vi "V_Estados.vi"() -> ()   [LabVIEW 2022 SP3]
uses:
  <vilib>/imath/engines/lvmath2/RunTimeEngine/Managers/WorkSpace/UID Generator.vi
  <vilib>/imath/engines/lvmath2/RunTimeEngine/RunTimeType/NIMS_RunTimeType_From StrictType (excl LVString).vi
  <instcachedir>/0/NIMS_RunTimeType_From StrictType (excl LVString)_70DEE8F51B6B495C85F505DE4E7061F1.lvgen/NIMS_RunTimeType_From StrictType (excl LVString)_70DEE8F51B6B495C85F505DE4E7061F1_000.vi
  <vilib>/imath/engines/lvmath2/RunTimeEngine/LocalVariableDefStatement/MC_LocalVariableDefStatement_Display.vi
  <vilib>/imath/engines/lvmath2/RunTimeEngine/VariableToken/NIMS_VariableToken_CondDefined.vi
  <instcachedir>/0/NIMS_VariableToken_CondDefined_190C34D11DD44198A50DB545329B6163.lvgen/NIMS_VariableToken_CondDefined_190C34D11DD44198A50DB545329B6163_003.vi
  <vilib>/imath/engines/lvmath2/RunTimeEngine/BuiltInFunctions/tf_to_ss/NIMS_tf_to_ss.vi
  <vilib>/imath/engines/lvmath2/RunTimeEngine/ErrorHandling/NIMS_Create Error From Enums.vi
  <vilib>/imath/engines/lvmath2/RunTimeEngine/BuiltInFunctions/transpose/NIMS_transpose(GM).vi
  <instcachedir>/0/NIMS_transpose(GM)_822C4B39CC3F4B34B360A85316D387F1.lvgen/NIMS_transpose(GM)_822C4B39CC3F4B34B360A85316D387F1_004.vi
  <vilib>/imath/engines/lvmath/Plug In/Control Design/BuiltInFunctions/obsvmx/NIMS_CD_obsvmx(A,B).vi
  <vilib>/imath/engines/lvmath/Plug In/Control Design/BuiltInFunctions/ctrbmx/NIMS_CD_ctrbmx(A,B).vi
  <vilib>/imath/engines/lvmath2/RunTimeEngine/BuiltInFunctions/rank/NIMS_rank.vi
  <instcachedir>/0/NIMS_rank_39A1B4AED7134F5694149EE328E336E6.lvgen/NIMS_rank_39A1B4AED7134F5694149EE328E336E6_000.vi
  <vilib>/imath/engines/lvmath2/RunTimeEngine/ErrorHandling/NIMS_Error From Error Code.vi
  <vilib>/imath/engines/lvmath2/RunTimeEngine/BuiltInFunctions/det/NIMS_det.vi
  <instcachedir>/0/NIMS_det_FC43403F6A814B2FA6A2876A6DC65E99.lvgen/NIMS_det_FC43403F6A814B2FA6A2876A6DC65E99_000.vi
  <vilib>/imath/engines/lvmath/Plug In/Control Design/BuiltInFunctions/ss/NIMS_CD_ss(A,B,C,D).vi
  <instcachedir>/0/NIMS_RunTimeType_From StrictType (excl LVString)_70DEE8F51B6B495C85F505DE4E7061F1.lvgen/NIMS_RunTimeType_From StrictType (excl LVString)_70DEE8F51B6B495C85F505DE4E7061F1_032.vi
  <vilib>/imath/engines/lvmath/Plug In/Control Design/BuiltInFunctions/step/NIMS_CD_[Y,T,X]=step(SS,[Tinfo]).vi
  <vilib>/imath/engines/lvmath2/RunTimeEngine/BuiltInFunctions/inv/NIMS_inv(GM).vi
  <instcachedir>/0/NIMS_inv(GM)_A6DF8FE880224208AACFE4CF9F659502.lvgen/NIMS_inv(GM)_A6DF8FE880224208AACFE4CF9F659502_000.vi
  <vilib>/imath/engines/lvmath2/RunTimeEngine/BuiltInFunctions/size/NIMS_I32Row=size(GM).vi
  <instcachedir>/0/NIMS_I32Row=size(GM)_10ACDCB9F1F84A7E9F42C91D87611FB5.lvgen/NIMS_I32Row=size(GM)_10ACDCB9F1F84A7E9F42C91D87611FB5_001.vi
  <vilib>/imath/engines/lvmath2/RunTimeEngine/IndexRead/NIMS V(S).vi
  <instcachedir>/0/NIMS V(S)_0488751826AF41519A22953C041130DC.lvgen/NIMS V(S)_0488751826AF41519A22953C041130DC_002.vi
  <vilib>/imathl/engines/lvmath/Functions/Error Handling/Create Error.vi
  <instcachedir>/0/NIMS_VariableToken_CondDefined_190C34D11DD44198A50DB545329B6163.lvgen/NIMS_VariableToken_CondDefined_190C34D11DD44198A50DB545329B6163_001.vi
  <instcachedir>/0/NIMS_VariableToken_CondDefined_190C34D11DD44198A50DB545329B6163.lvgen/NIMS_VariableToken_CondDefined_190C34D11DD44198A50DB545329B6163_005.vi
  <instcachedir>/0/NIMS_VariableToken_CondDefined_190C34D11DD44198A50DB545329B6163.lvgen/NIMS_VariableToken_CondDefined_190C34D11DD44198A50DB545329B6163_004.vi
  <vilib>/imath/engines/lvmath/Functions/Error Handling/MergeErrorsWrapper.vi
  <vilib>/imath/engines/lvmath2/RunTimeEngine/Managers/SymbolTable/Clear UID.vi
  <vilib>/imath/engines/lvmath2/RunTimeEngine/NodeEndStatement/NIMS_NodeEndStatement_Output.vi
  <instcachedir>/0/NIMS_NodeEndStatement_Output_53EC0D466D134D7ABD903AC30B43404B.lvgen/NIMS_NodeEndStatement_Output_53EC0D466D134D7ABD903AC30B43404B_009.vi
  <instcachedir>/0/NIMS_NodeEndStatement_Output_53EC0D466D134D7ABD903AC30B43404B.lvgen/NIMS_NodeEndStatement_Output_53EC0D466D134D7ABD903AC30B43404B_002.vi
  <instcachedir>/0/NIMS_NodeEndStatement_Output_53EC0D466D134D7ABD903AC30B43404B.lvgen/NIMS_NodeEndStatement_Output_53EC0D466D134D7ABD903AC30B43404B_001.vi
  <vilib>/imath/engines/lvmath2/RunTimeEngine/ErrorHandling/NIMS_Finalize Error.vi
  <vilib>/imath/engines/lvmath2/RunTimeEngine/Managers/SymbolTable/NIMS_WorkSpace.lvlib
panel:
  out "Observabilidad":string="El Sistema es Controlabe"
  out "Controlabilidas":string="El Sistema es Controlabe"
  out "Ta_Mo":i32
  out "Ta_Mc":i32
  out "GRAFICA":dbl[][](graph)
  out "Dete_MO":dbl
  out "Dete_MC":dbl
  out "Rango_MO":i32
  out "Rango_MC":i32
  out "MC":dbl[][](array[numeric])
  out "MO":dbl[][](array[numeric])
  out "CO":dbl[][](array[numeric])
  out "BO":dbl[][](array[numeric])
  out "AO":dbl[][](array[numeric])
  out "C":dbl[][](array[numeric])
  out "B":dbl[][](array[numeric])
  out "A":dbl[][](array[numeric])
  in  "ORDEN":dbl
  in  "Stop":bool
  in  "b4":dbl
  in  "a4":dbl
  in  "b3":dbl
  in  "a2":dbl
  in  "b2":dbl
  in  "b1":dbl
  in  "b0":dbl
  in  "a1":dbl
  in  "a3":dbl
  # "+"
  # "z^-1  +"
  # "z^-2  +"
  # "z^-3  +"
  # "z^-4"
  # "Y(z)"
  # "G(Z)="
  # "="
  # "U(z)"
  # "1  +"
  # "z^-1  +"
  # "z^-2  +"
  # "z^-3  +"
  # "z^-4"
  # "FORMA CANONICA CONTROLABLE"
  # "FORMA CANONICA OBSERVABLE"
  # "CONTROLABILIDAD Y OBSERVABILIDAD DEL SISTEMA"
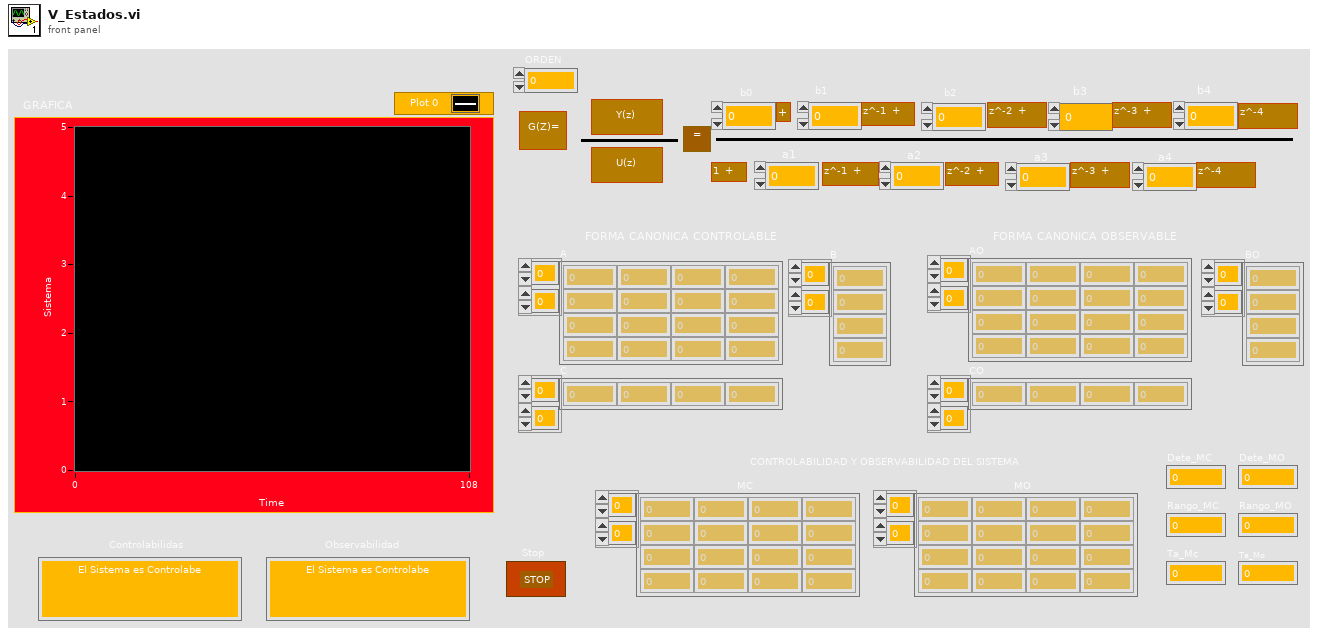
[diagram p1: front panel]
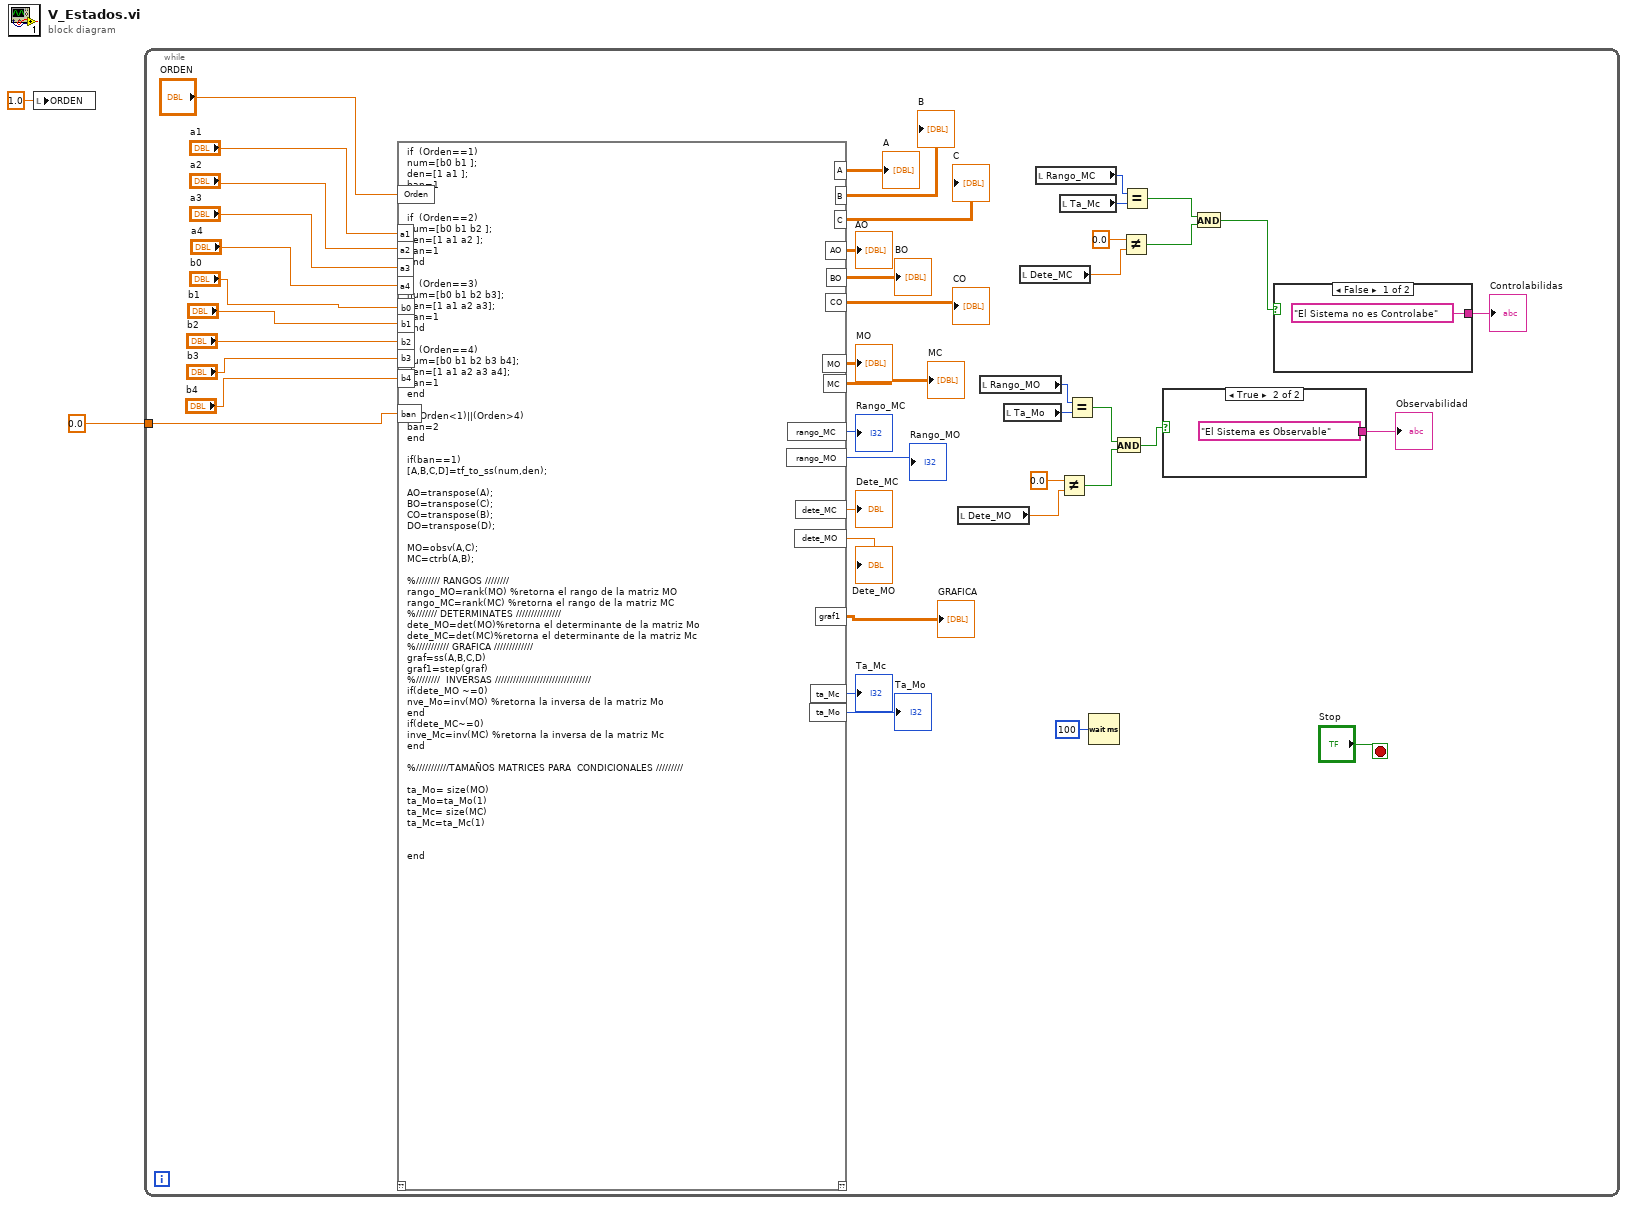
[diagram p0: block diagram]
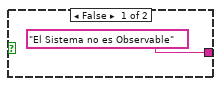
[diagram p2: hidden frame]
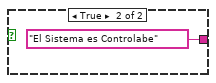
[diagram p3: hidden frame]
diagram:
  n1 = local write "ORDEN"(1.0 ("ORDEN")) -> ()
  n2 = while {
    tunnel: 0.0 ("ban") -> [w14]
    stop <- "Stop" stop-if-true
    n3 = mathscript code="if  (Orden==1)\nnum=[b0 b1 ];\nden=[1 a1 ];\nban=1\nend \n\nif  (Orden==2)\nnum=[b0 b1 b2 ];\nden=[1 a1 a2 ];\nban=1\nend \n\nif  (Orden==3)\nnum=[b0 b1 b2 b3];\nden=[1 a1 a2 a3];\nban=1\nend \n\nif  (Orden==4)\nnum=[b0 b1 b2 b3 b4];\nden=[1 a1 a2 a3 a4];\nban=1\nend \n\nif (Orden<1)||(Orden>4)\nban=2\nend\n\nif(ban==1) \n[A,B,C,D]=tf_to_ss(num,den);\n\nAO=transpose(A);\nBO=transpose(C);\nCO=transpose(B);\nDO=transpose(D);\n\nMO=obsv(A,C);\nMC=ctrb(A,B);\n\n%//////// RANGOS ////////\nrango_MO=rank(MO) %retorna el rango de la matriz MO\nrango_MC=rank(MC) %retorna el rango de la matriz MC\n%/////// DETERMINATES ///////////////\ndete_MO=det(MO)%retorna el determinante de la matriz Mo\ndete_MC=det(MC)%retorna el determinante de la matriz Mc\n%/////////// GRAFICA /////////////\ngraf=ss(A,B,C,D)\ngraf1=step(graf)\n%////////  INVERSAS ////////////////////////////////\nif(dete_MO ~=0)\nnve_Mo=inv(MO) %retorna la inversa de la matriz Mo\nend\nif(dete_MC~=0)\ninve_Mc=inv(MC) %retorna la inversa de la matriz Mc\nend\n\n%///////////TAMAÑOS MATRICES PARA  CONDICIONALES /////////\n\nta_Mo= size(MO)\nta_Mo=ta_Mo(1)\nta_Mc= size(MC)\nta_Mc=ta_Mc(1)\n\n \nend"("a1"="a1", "a2"="a2", "a3"="a3", "a4"="a4", "b0"="b0", "b1"="b1", "b2"="b2", "b3"="b3", "b4"="b4", "Orden"="ORDEN", "ban"=w14) -> ("A"=→"A":dbl[][], "B"=→"B":dbl[][], "C"=→"C":dbl[][], "AO"=→"AO":dbl[][], "BO"=→"BO":dbl[][], "CO"=→"CO":dbl[][], "MO"=→"MO":dbl[][], "MC"=→"MC":dbl[][], "rango_MC"=→"Rango_MC":i32, "rango_MO"=→"Rango_MO":i32, "dete_MC"=→"Dete_MC":dbl, "dete_MO"=→"Dete_MO":dbl, "graf1"=→"GRAFICA":dbl[][], "ta_Mc"=→"Ta_Mc":i32, "ta_Mo"=→"Ta_Mo":i32)  [unwired: 1 in, 1 out]
    n4 = local read "Dete_MO"() -> (w6:dbl)
    n5 = local read "Rango_MO"() -> (w25:i32)
    n6 = local read "Ta_Mo"() -> (w24:i32)
    n7 = local read "Dete_MC"() -> (w8:dbl)
    n8 = local read "Rango_MC"() -> (w28:i32)
    n9 = Not Equal?(x=0.0, y=w6) -> (x != y?=w4:bool)
    n10 = local read "Ta_Mc"() -> (w27:i32)
    n11 = Equal?(x=w25, y=w24) -> (x = y?=w5:bool)
    n12 = Wait (ms)(milliseconds to wait=u32 100) -> ()  [unwired: 1 out]
    n13 = And(x=w5, y=w4) -> (x .and. y?=w3:bool)
    n14 = Not Equal?(x=0.0, y=w8) -> (x != y?=w10:bool)
    n15 = Equal?(x=w28, y=w27) -> (x = y?=w12:bool)
    n16 = case shown="True" w3 {
      tunnel: ["El Sistema no es Observable" "El Sistema es Observable"] -> w26
      frame False {
      }
      frame True {
      }
    }
    "Observabilidad" <- w26
    n17 = And(x=w12, y=w10) -> (x .and. y?=w11:bool)
    n18 = case shown="False" w11 {
      tunnel: ["El Sistema no es Controlabe" "El Sistema es Controlabe"] -> w29
      frame False {
      }
      frame True {
      }
    }
    "Controlabilidas" <- w29
  }
